vi "Add to Array if Not Present (I32).vi"(4 "I32":i32, 5 "I32 Array":i32[](array[numeric])) -> (1 "New I32 Array":i32[](array[numeric]))   [LabVIEW 2011]
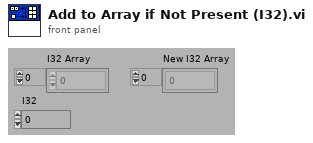
[diagram p1: front panel]
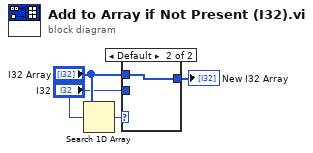
[diagram p0: block diagram]
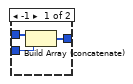
[diagram p2: hidden frame]
diagram:
  n1 = Search 1D Array(1D array="I32 Array", element="I32") -> (index of element=w4:i32)  [unwired: 1 out]
  n2 = case shown="Default" w4 {
    tunnel: "I32 Array" -> [w7 w8]
    tunnel: "I32" -> [w6 _]
    tunnel: [w5 w8] -> w1
    frame -1 {
      n3 = Build Array (concatenate)(w7, w6) -> (w5:i32[])
    }
    frame Default {
    }
  }
  "New I32 Array" <- w1
